vi "Set Close Panel (Yes or No).vi"(0 "reference in":refnum<class "Generic Utilities.lvclass">, 5 "error in (no error)":errorcluster, 6 "Front Panel Window:Show Menu Bar":bool=TRUE) -> (14 "reference out":refnum<class "Generic Utilities.lvclass">, 19 "error out":errorcluster)   [LabVIEW 2022 SP3, in "Generic Utilities.lvclass"]
uses:
  Generic Utilities.lvclass
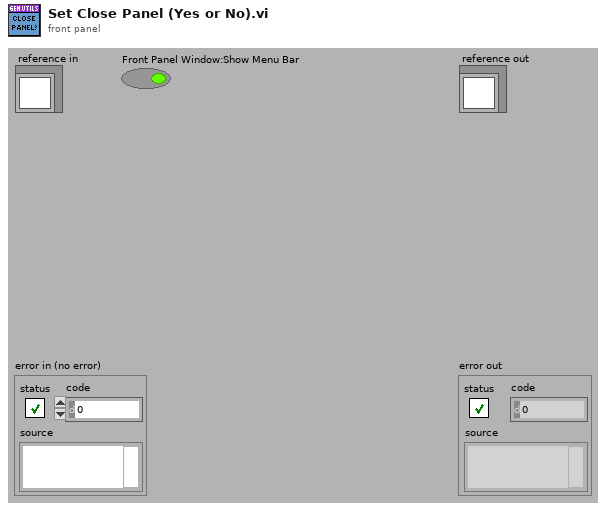
[diagram p1: front panel]
types:
  T1 = enum16{"Always On", "Always Off", "Off While Running"}
  T2 = enum32{"invalid app kind", "Development System", "Run Time System", "Student Edition", "Embedded LabVIEW", "Evaluation", "Custom"}
  T3 = typedef "Generic Utilities.lvclass/ObjectAttributesRef.ctl" = refnum<data-value>
  T4 = typedef "Generic Utilities.lvclass/ObjectAttributes.ctl" = cluster{"GUI Parameters":T5, "State Machine Control":cluster{"Timeout":i32, "State Queue":string[], "State History":string[], "State History Length":i32}, "Logging File Path":path, "OBJ not a refnum?":bool, "Timer Start":timestamp, "FP Refnums":T6}
  T5 = typedef "Generic Utilities.lvclass/GUI Parameters.ctl" = cluster{"Application Name":string, "GUI VI Ref":refnum<vi>, "Close Panel?":bool, "Message Window ref":refnum<vi>, "Version #":string}
  T6 = typedef "Generic Utilities.lvclass/FP Refnums.ctl" = cluster{"Panel refnum":refnum<vi>, "Control Labels":string[], "Refnums":refnum<vi>[]}
  T7 = enum32{"Invalid", "Standard", "Closed", "Hidden", "Minimized", "Maximized"}
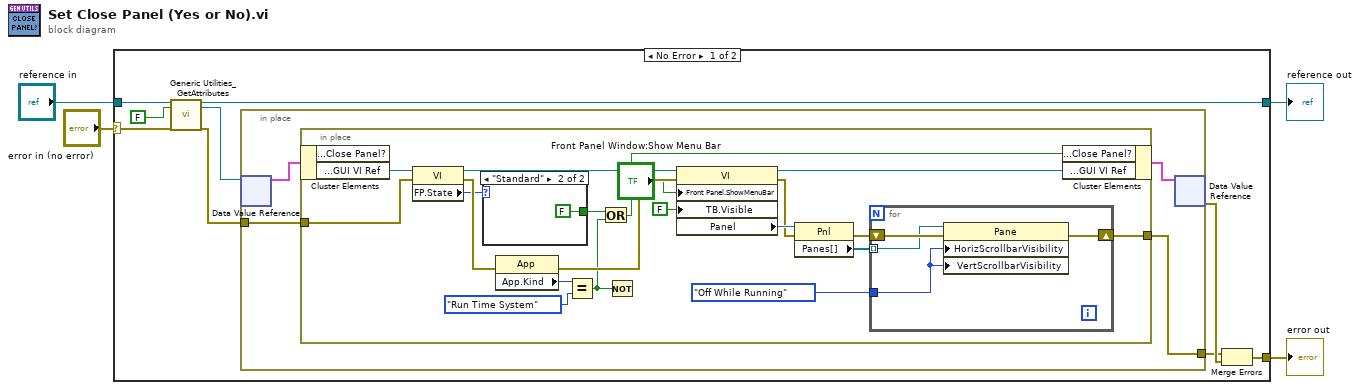
[diagram p0: block diagram]
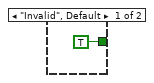
[diagram p2: hidden frame]
diagram:
  n1 = case shown="No Error" "error in (no error)" {
    selector: "error in (no error)" -> [w8 w45]
    tunnel: [w13 w45] -> w3
    tunnel: [w7 w44] -> w1
    tunnel: "reference in" -> [w10 w44]
    frame No Error {
      n2 = call "Generic Utilities_GetAttributes.vi"("reference in"=w10, "return data? (T)"=FALSE, "error in (no error)"=w8) -> ("reference out"=w7:refnum<class "Generic Utilities.lvclass">, "attributes ref"=w6:T3, "error out"=w5:errorcluster)  [unwired: 13 in, 1 out]
      n3 = in-place {
        in-place-border: [w14] -> w11
        in-place-border: w5 -> [w15]
        n4 = in-place-dvr #1(w6) -> (w16:T4)  [unwired: 1 out]
        n5 = in-place {
          in-place-border: w15 -> [w35]
          in-place-border: [w22] -> w14
          n6 = in-place-cluster #2(w16) -> ("GUI Parameters.GUI VI Ref"=w33:refnum<vi>)  [unwired: 1 out]
          n7 = property class="VI"(reference=w33, error in=w35) -> (reference out=w30:refnum<vi>, error out=w34:errorcluster, "FP.State"=w32:T7)
          n8 = case shown="\"Standard\"" w32 {
            tunnel: [TRUE FALSE] -> w31
            frame "Invalid", Default {
            }
            frame "Standard" {
            }
          }
          n9 = property class="App"(error in=w34) -> (error out=w27:errorcluster, "App.Kind"=w36:T2)  [unwired: 1 in, 1 out]
          n10 = Equal?(x=w36, y=T2."Run Time System" ("Application:Kind")) -> (x = y?=w21:bool)
          n11 = Or(x=w31, y=w21) -> (x .or. y?=w29:bool)
          n12 = Not(x=w21) -> ()  [unwired: 1 out]
          n13 = property class="VI"(reference=w30, error in=w27, "Front Panel.ShowMenuBar"="Front Panel Window:Show Menu Bar", "TB.Visible"=FALSE ("Tool Bar:Visible")) -> (reference out=w28:refnum<vi>, error out=w25:errorcluster, "Panel"=w26:refnum<vi>)
          n14 = property class="Pnl"(reference=w26, error in=w25) -> (error out=w24:errorcluster, "Panes[]"=w23:refnum<vi>[])  [unwired: 1 out]
          n15 = for {
            shift-right: [w40] -> w22
            shift-left: w24 -> [w41]
            tunnel: w23 -> [w39] mode=indexing
            tunnel: T1."Off While Running" ("Horizontal Scrollbar Visibility") -> [w38]
            n16 = property class="Pane"(reference=w39, error in=w41, "HorizScrollbarVisibility"=w38, "VertScrollbarVisibility"=w38) -> (error out=w40:errorcluster)  [unwired: 1 out]
          }
          n17 = in-place-cluster #2("GUI Parameters.Close Panel?"=w29, "GUI Parameters.GUI VI Ref"=w28) -> (w17:T4)
        }
        n18 = in-place-dvr #1(w17) -> (w12:errorcluster)  [unwired: 1 out]
      }
      n19 = Merge Errors(w11, w12) -> (w13:errorcluster)
    }
    frame Error {
    }
  }
  "error out" <- w3
  "reference out" <- w1
